vi "dataset.add.vi"(6 "Series Tags":map{string, string}(c390), 8 "error in":errorcluster, 9 "dataset":refnum<class "dataset.lvclass">, 10 "Datascope Name":string, 11 "asset in":refnum<class "asset.lvclass">) -> (0 "error out":errorcluster, 3 "asset out":refnum<class "asset.lvclass">)   [LabVIEW 2020, in "asset.lvclass"]
uses:
  asset.lvclass
  datasources/dataset/dataset.lvclass
  asset.lvclass/asset.ctl
  Nominal Client/Nominal Client.lvclass/Nominal Client.ctl
  nominal types/workspace/workspace.lvclass/workspace.ctl
  Nominal Client/workspace.get.vi
  <vilib>/JDP Science/JSONtext/Merge into Object.vi
  Nominal Client/workspace.add_to_payload.vi/88650e10-de3e-481c-85db-71cb0fdf4485.vi
  nominal types/workspace/rid.get.vi
  <vilib>/JDP Science/JSONtext/Variant to JSON Text.vi
  <vilib>/JDP Science/JSONtext/Get all Object Items.vi
  <vilib>/JDP Science/JSONtext/Set Multiple Object Items.vi
  <vilib>/JDP Science/JSONtext/LVClass Serializer/JSONtext LVClass Serializer.lvclass
  Nominal Client/Nominal Client.lvclass
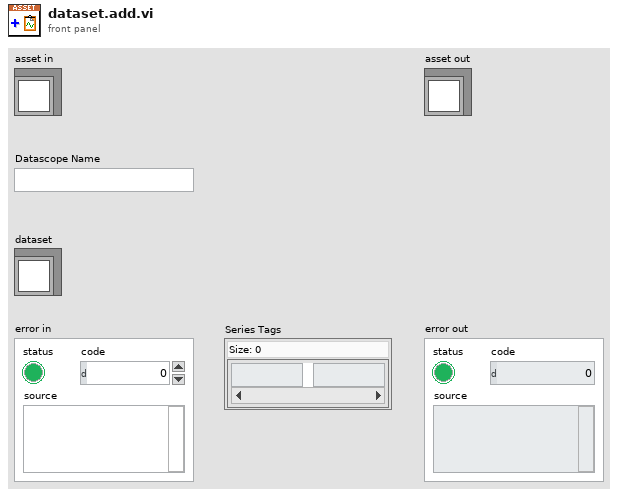
[diagram p1: front panel]
types:
  T1 = typedef "dataScopes.lvlib/links.ctl" = cluster{"URL":string, "Title":string}[]
  T2 = typedef "dataScopes.lvlib/data_scopes.ctl" = T3[]
  T3 = typedef "dataScopes.lvlib/data_scope.ctl" = cluster{"dataScopeName":string, "dataSource":T4, "seriesTags":map{string, string}, "offset":T6}
  T4 = typedef "dataScopes.lvlib/data_source.ctl" = cluster{"type":T5, "rid":string}
  T5 = typedef "dataScopes.lvlib/type.ctl" = enum16{"dataset", "connection", "logSet", "video"}
  T6 = typedef "dataScopes.lvlib/offset.ctl" = cluster{"seconds":i32, "nanos":i32, "picos":i32}
  T7 = cluster{"rid":string, "title":string, "properties":refnum<class "properties.lvclass">, "labels":refnum<class "labels.lvclass">, "Links":T1, "datascopes":T2, "createdAt":timestamp, "updatedAt":timestamp, "attachments":refnum<class "labels.lvclass">, "isStaged":bool, "isArchived":bool, "description":string, "createdBy":string, "type":string}
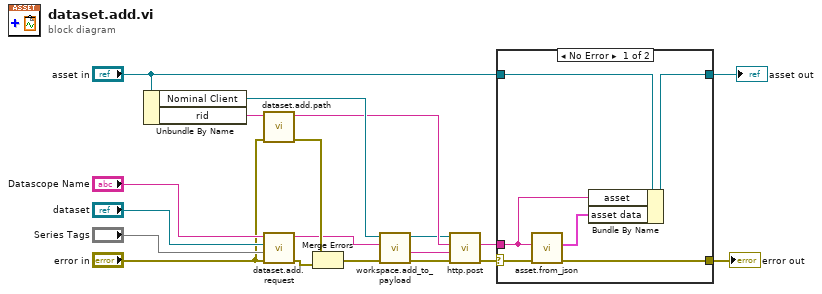
[diagram p0: block diagram]
diagram:
  n1 = Unbundle By Name("asset in") -> ("Nominal Client"=w10:refnum<class "Nominal Client.lvclass">, "rid"=w13:string)
  n2 = call "dataset.add.path.vi"("error in"="error in", "Asset RID"=w13) -> ("error out"=w11:errorcluster, "Path"=w2:string)  [unwired: 8 in]
  n3 = call "dataset.add.request.vi"("error in"="error in", "Series Tags"="Series Tags", "dataset"="dataset", "DataScope Name"="Datascope Name") -> ("error out"=w8:errorcluster, "Request"=w9:string)  [unwired: 6 in]
  n4 = Merge Errors(w11, w8) -> (w7:errorcluster)
  n5 = call "workspace.add_to_payload.vi"("error in"=w7, "JSON payload in"=w9, "Nominal Client in"=w10) -> ("error out"=w5:errorcluster, "JSON payload out"=w6:string, "Nominal Client out"=w1:refnum<class "Nominal Client.lvclass">)  [unwired: 6 in]
  n6 = call "http.post.vi"("error in"=w5, "Request body"=w6, "Path"=w2, "Nominal Client in"=w1) -> ("error out"=w4:errorcluster, "Response"=w3:string)  [unwired: 4 in, 2 out]
  n7 = case shown="No Error" w4 {
    selector: w4 -> [w25 w27]
    tunnel: [w24 w27] -> w19
    tunnel: "asset in" -> [w23 w26]
    tunnel: w3 -> [w21 _]
    tunnel: [w20 w26] -> w17
    frame No Error {
      n8 = call "asset.from_json.vi"("error in"=w25, "asset"=w21) -> ("error out"=w24:errorcluster, "Asset Data"=w22:T7)  [unwired: 8 in]
      n9 = Bundle By Name(cluster=w23, "asset"=w21, "asset data"=w22) -> (w20:refnum<class "asset.lvclass">)
    }
    frame Error {
    }
  }
  "asset out" <- w17
  "error out" <- w19
